vi "statistics Sender to SSLView UDP TX.vi"(7 "Statistics":T1, 8 "Port:":u16=20011, 9 "SSL Vision Address:":string="127.0.0.1", 10 "isteamyellow":bool=TRUE, 11 "Robots":T5[](array[typedef])) -> ()   [LabVIEW 2017]
uses:
  grSim/grSim Robot Command.ctl
  grSim/grSim RobotReplacement.ctl
  grSim/grSim_BallReplacement.ctl
  <extravilib>/ChannelInstances/Lossy Stream-a[.](i32)/)Channel.ctl
  <extravilib>/ChannelInstances/Lossy Stream-a[.](i32).lvlib
panel:
  in  "grSim replacement":T4={"grSim_RobotReplacement"=[{"x"=0.0, "y"=-450.0, "dir"=0.0, "yellowteam"=FALSE, "id"=0}, {"x"=0.0, "y"=-270.0, "dir"=0.0, "yellowteam"=FALSE, "id"=1}, {"x"=0.0, "y"=-90.0, "dir"=0.0, "yellowteam"=FALSE, "id"=2}, {"x"=0.0, "y"=90.0, "dir"=0.0, "yellowteam"=FALSE, "id"=3}, {"x"=0.0, "y"=270.0, "dir"=0.0, "yellowteam"=FALSE, "id"=4}, {"x"=0.0, "y"=450.0, "dir"=0.0, "yellowteam"=FALSE, "id"=5}], "grSim_BallReplacement"={"x"=0.0, "y"=0.0, "vx"=0.0, "vy"=0.0}}
  out "error out":errorcluster
  out "Array":u8[](array[numeric]) format="%02x"
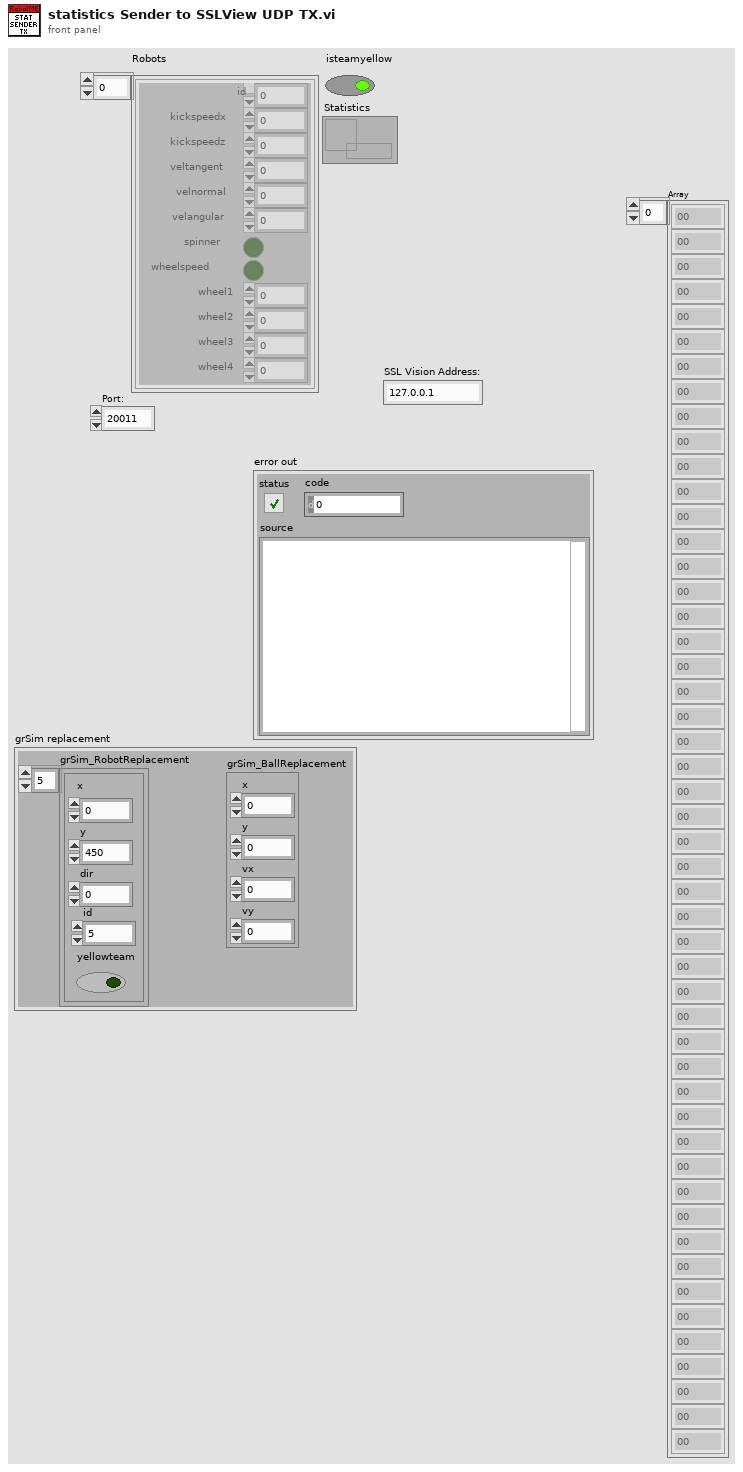
[diagram p1: front panel]
types:
  T1 = typedef "Lossy Stream-a[.](i32).lvlib/)Channel.ctl" = refnum<queue>
  T2 = typedef "grSim RobotReplacement.ctl" = cluster{"x":dbl, "y":dbl, "dir":dbl, "yellowteam":bool, "id":u32}
  T3 = typedef "grSim_BallReplacement.ctl" = cluster{"x":dbl, "y":dbl, "vx":dbl, "vy":dbl}
  T4 = cluster{"grSim_RobotReplacement":T2[], "grSim_BallReplacement":T3}
  T5 = typedef "grSim Robot Command.ctl" = cluster{"id":u32, "kickspeedx":sgl, "kickspeedz":sgl, "veltangent":sgl, "velnormal":sgl, "velangular":sgl, "spinner":bool, "wheelspeed":bool, "wheel1":sgl, "wheel2":sgl, "wheel3":sgl, "wheel4":sgl}
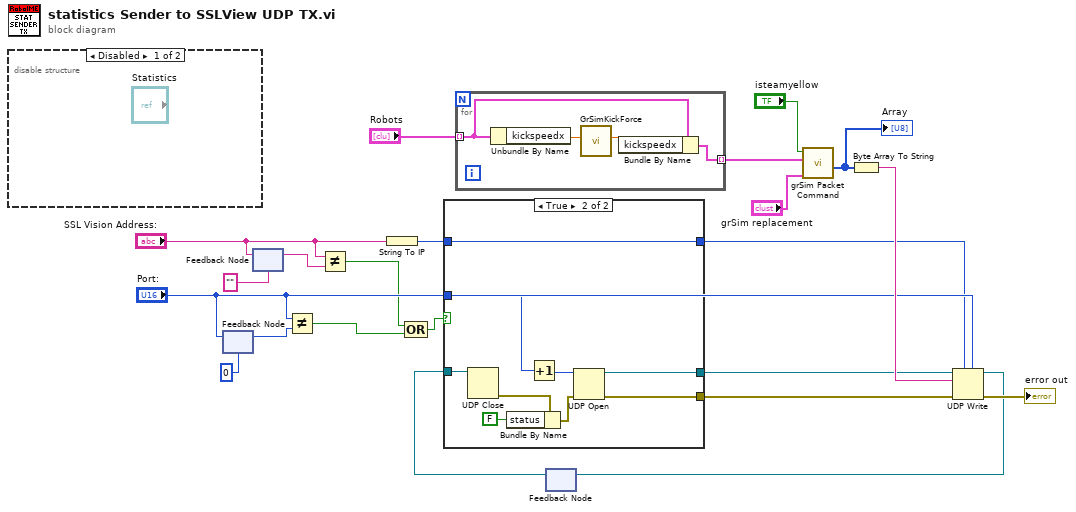
[diagram p0: block diagram]
diagram:
  n1 = disable-structure shown="Disabled" {
    frame Disabled {
    }
    frame Enabled {
    }
  }
  n2 = feedback #1(u16 0 ("Port:")) -> (w18:u16)
  n3 = feedback-in #1("Port:") -> ()
  n4 = feedback #2("" ("SSL Vision Address:")) -> (w16:string)
  n5 = feedback-in #2("SSL Vision Address:") -> ()
  n6 = Not Equal?(x="Port:", y=w18) -> (x != y?=w14:bool)
  n7 = Not Equal?(x="SSL Vision Address:", y=w16) -> (x != y?=w15:bool)
  n8 = String To IP(1:"SSL Vision Address:") -> (0:w5:u32)
  n9 = Compound Arithmetic op=OR(w15, w14) -> (w13:bool)
  n10 = for {
    tunnel: "Robots" -> [w27] mode=indexing
    tunnel: [w26] -> w2 mode=indexing
    n11 = Unbundle By Name(w27) -> ("kickspeedx"=w25:sgl)
    n12 = call "GrSimKickForce.vi"("real kick"=w25) -> ("grsim kick"=w24:dbl)  [unwired: 10 in]
    n13 = Bundle By Name(cluster=w27, "kickspeedx"=w24) -> (w26:T5)
  }
  n14 = feedback #3() -> (w11:refnum<k16>)  [unwired: 1 in]
  n15 = case shown="True" w13 {
    tunnel: [_ w38] -> w19
    tunnel: [w29 w36] -> w10
    tunnel: "Port:" -> [_ w35]
    tunnel: w5 -> [w28 w33]
    tunnel: w11 -> [w29 w34]
    tunnel: [w28 w33] -> w4
    frame False {
    }
    frame True {
      n16 = UDP Close(connection ID=w34) -> (error out=w32:errorcluster)  [unwired: 1 in, 1 out]
      n17 = Bundle By Name(cluster=w32, "status"=FALSE) -> (w31:errorcluster)
      n18 = Increment(x=w35) -> (x+1=w37:u16)
      n19 = UDP Open(8:w31, 11:w37) -> (port=w36:refnum<k16>, 0:w38:errorcluster)  [unwired: 3 in, 1 out]
    }
  }
  n20 = call "grSim Packet Command.vi"("grSim replacement"="grSim replacement", "Robots"=w2, "isteamyellow"="isteamyellow") -> ("Array"=w21:u8[])  [unwired: 8 in]
  "Array" <- w21
  n21 = Byte Array To String(unsigned byte array=w21) -> (string=w20:string)
  n22 = UDP Write(address=w4, port or service name="Port:", connection ID=w10, data in=w20, 8:w19) -> (error out=→"error out":errorcluster, 3:w9:refnum<k16>)  [unwired: 1 in]
  n23 = feedback-in #3(w9) -> ()
